vi "TombOfTheMask.vi"() -> ()   [LabVIEW 2014]
panel:
  out "stage":dbl
  in  "start":cluster{"String":string, "play":bool}={"String"="\nTomb Of The Mask", "play"=FALSE}
  in  "quit":bool
  in  "next stage or choosing stage":T1
  in  "choosing stage":T2
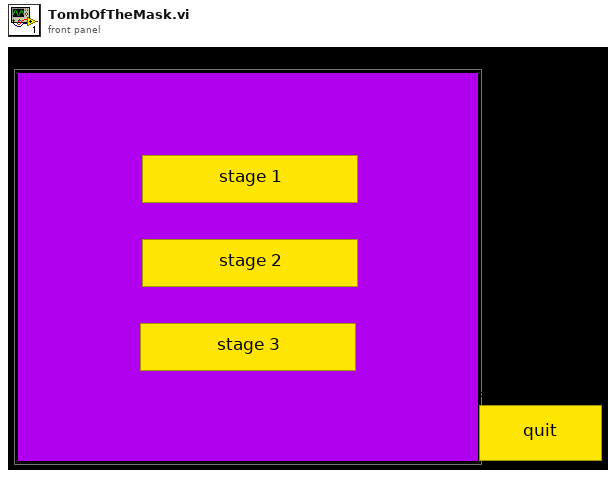
[diagram p1: front panel]
types:
  T1 = cluster{"next stage ":bool, "back":bool, "Boolean":bool, "Boolean 2":bool, "Boolean 3":bool}
  T2 = cluster{"stage 1":bool, "stage 2":bool, "stsage 3":bool}
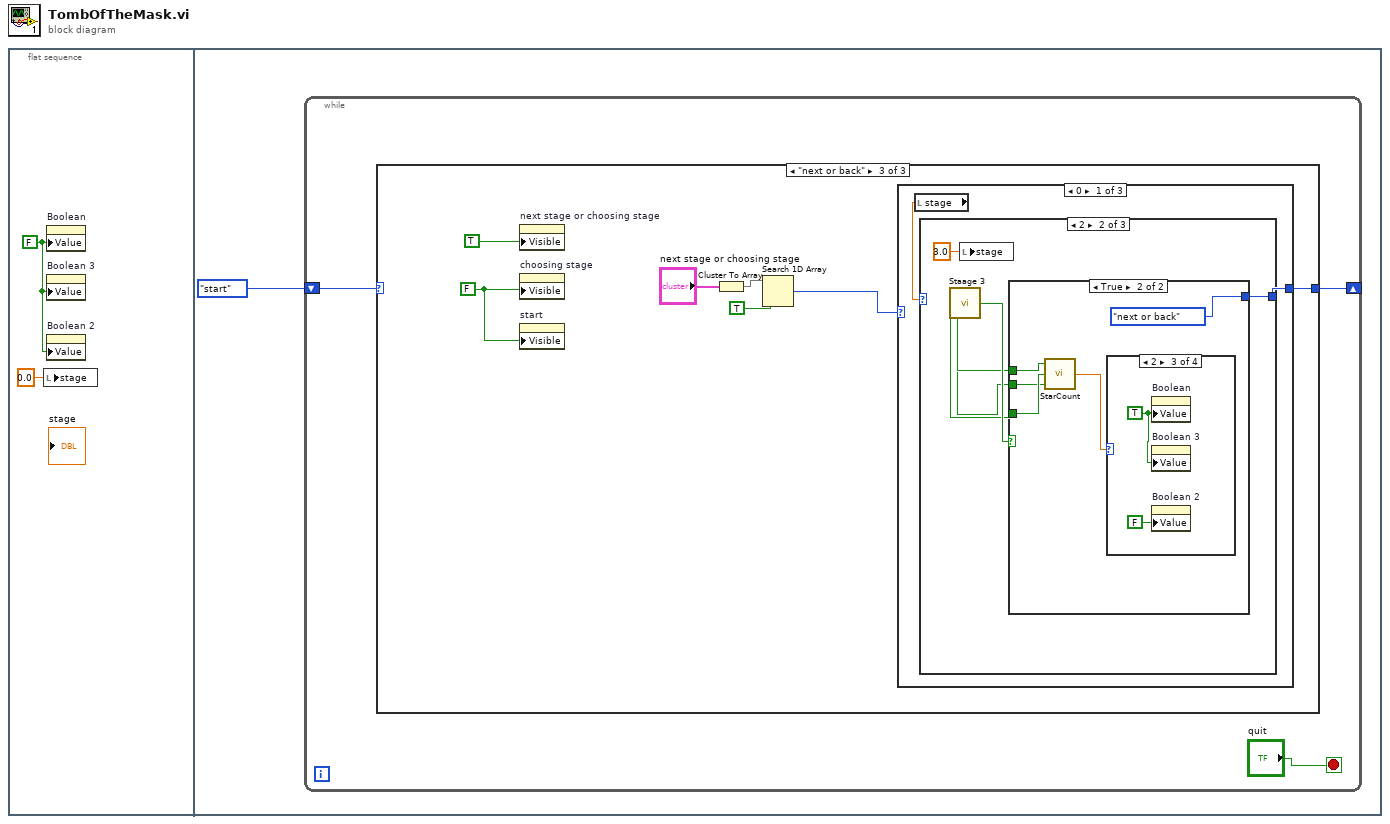
[diagram p0: block diagram]
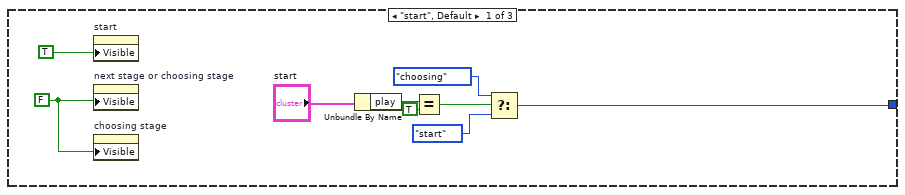
[diagram p2: hidden frame]
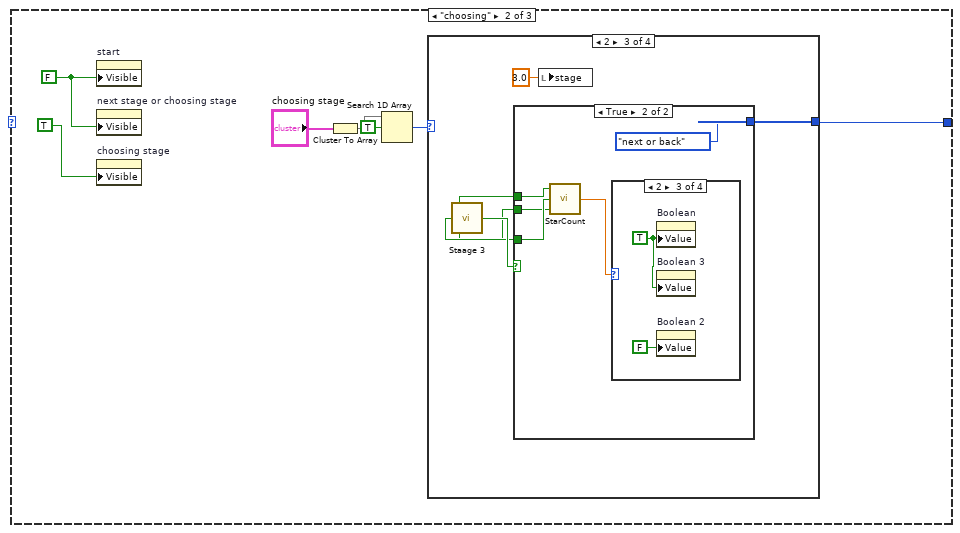
[diagram p3: hidden frame]
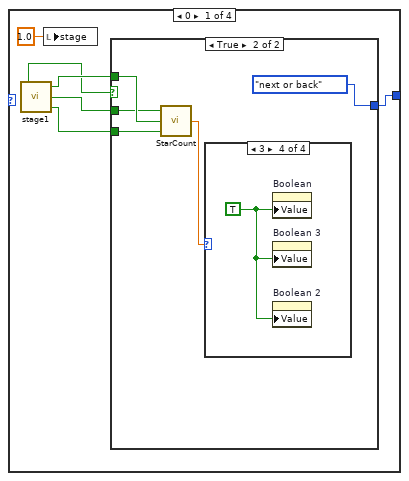
[diagram p4: hidden frame]
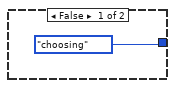
[diagram p5: hidden frame]
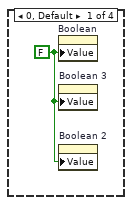
[diagram p6: hidden frame]
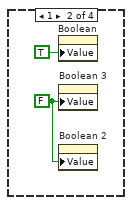
[diagram p7: hidden frame]
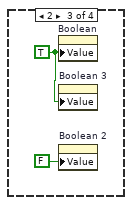
[diagram p8: hidden frame]
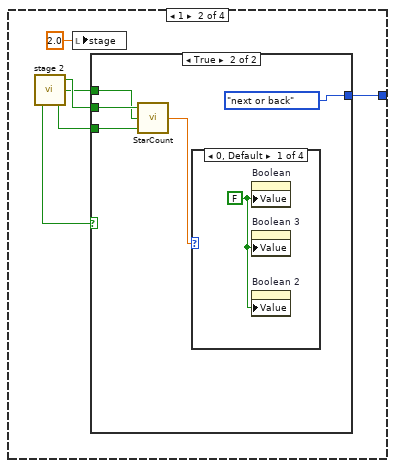
[diagram p9: hidden frame]
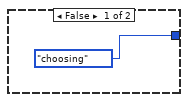
[diagram p10: hidden frame]
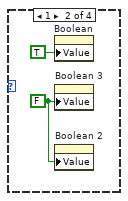
[diagram p11: hidden frame]
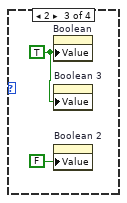
[diagram p12: hidden frame]
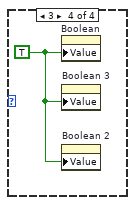
[diagram p13: hidden frame]
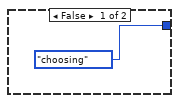
[diagram p14: hidden frame]
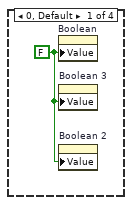
[diagram p15: hidden frame]
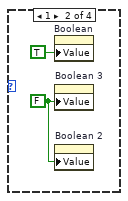
[diagram p16: hidden frame]
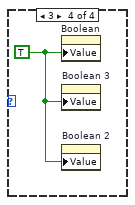
[diagram p17: hidden frame]
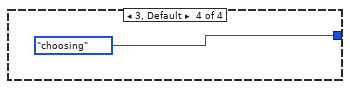
[diagram p18: hidden frame]
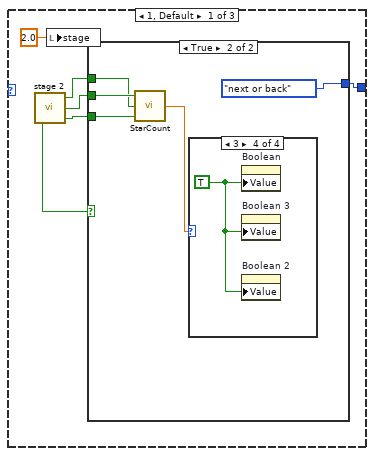
[diagram p19: hidden frame]
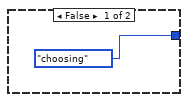
[diagram p20: hidden frame]
diagram:
  n1 = flat-sequence {
    frame #0 {
      w1 = FALSE ("Value")
      n2 = local write "stage"(0.0 ("stage")) -> ()
      n3 = property on="Boolean" class="Bool (strict)"("Value"=w1) -> ()  [unwired: 2 in, 2 out]
      n4 = property on="Boolean 3" class="Bool (strict)"("Value"=w1) -> ()  [unwired: 2 in, 2 out]
      n5 = property on="Boolean 2" class="Bool (strict)"("Value"=w1) -> ()  [unwired: 2 in, 2 out]
    }
    frame #1 {
      n6 = while {
        shift-right: [w5] -> _
        shift-left: enum16{"next or back", "choosing", "start"}."start" ("Enum") -> [w6]
        stop <- "quit" stop-if-true
        n7 = case shown="\"next or back\"" w6 {
          tunnel: [w7 w16 w78] -> w5
          frame "start", Default {
            w14 = FALSE ("Visible")
            n8 = property on="start" class="Clust"("Visible"=TRUE) -> ()  [unwired: 2 in, 2 out]
            n9 = property on="next stage or choosing stage" class="Clust"("Visible"=w14) -> ()  [unwired: 2 in, 2 out]
            n10 = property on="choosing stage" class="Clust"("Visible"=w14) -> ()  [unwired: 2 in, 2 out]
            n11 = Unbundle By Name("start") -> ("play"=w12:bool)
            n12 = Equal?(x=w12, y=TRUE) -> (x = y?=w10:bool)
            n13 = Select(t=enum16{"next or back", "choosing", "start"}."choosing" ("Enum"), s=w10, f=enum16{"next or back", "choosing", "start"}."start" ("Enum")) -> (s? t:f=w7:enum16{"next or back", "choosing", "start"})
          }
          frame "choosing" {
            w21 = FALSE ("Visible")
            n14 = property on="start" class="Clust"("Visible"=w21) -> ()  [unwired: 2 in, 2 out]
            n15 = property on="next stage or choosing stage" class="Clust"("Visible"=w21) -> ()  [unwired: 2 in, 2 out]
            n16 = property on="choosing stage" class="Clust"("Visible"=TRUE) -> ()  [unwired: 2 in, 2 out]
            n17 = Cluster To Array(cluster="choosing stage") -> (array=w19:bool[])
            n18 = Search 1D Array(1D array=w19, element=TRUE) -> (index of element=w17:i32)  [unwired: 1 in]
            n19 = case shown="2" w17 {
              tunnel: [w25 w41 w59 enum16{"next or back", "choosing", "start"}."choosing" ("Enum")] -> w16
              frame 0 {
                n20 = call "stage1.vi"() -> ("pass"=w24:bool, "Boolean 5"=w26:bool, "Boolean 8"=w23:bool, "Boolean 7"=w27:bool)
                n21 = local write "stage"(1.0 ("stage")) -> ()
                n22 = case shown="True" w24 {
                  tunnel: w27 -> [_ w34]
                  tunnel: w26 -> [_ w33]
                  tunnel: w23 -> [_ w32]
                  tunnel: [enum16{"next or back", "choosing", "start"}."choosing" ("Enum") enum16{"next or back", "choosing", "start"}."next or back" ("Enum")] -> w25
                  frame False {
                  }
                  frame True {
                    n23 = call "StarCount.vi"("Boolean 2"=w34, "Boolean"=w33, "Boolean 3"=w32) -> ("Numeric"=w30:dbl)
                    n24 = case shown="3" w30 {
                      frame 0, Default {
                        w35 = FALSE ("Value")
                        n25 = property on="Boolean" class="Bool (strict)"("Value"=w35) -> ()  [unwired: 2 in, 2 out]
                        n26 = property on="Boolean 3" class="Bool (strict)"("Value"=w35) -> ()  [unwired: 2 in, 2 out]
                        n27 = property on="Boolean 2" class="Bool (strict)"("Value"=w35) -> ()  [unwired: 2 in, 2 out]
                      }
                      frame 1 {
                        w36 = FALSE ("Value")
                        n28 = property on="Boolean" class="Bool (strict)"("Value"=TRUE) -> ()  [unwired: 2 in, 2 out]
                        n29 = property on="Boolean 3" class="Bool (strict)"("Value"=w36) -> ()  [unwired: 2 in, 2 out]
                        n30 = property on="Boolean 2" class="Bool (strict)"("Value"=w36) -> ()  [unwired: 2 in, 2 out]
                      }
                      frame 2 {
                        w39 = TRUE ("Value")
                        n31 = property on="Boolean" class="Bool (strict)"("Value"=w39) -> ()  [unwired: 2 in, 2 out]
                        n32 = property on="Boolean 3" class="Bool (strict)"("Value"=w39) -> ()  [unwired: 2 in, 2 out]
                        n33 = property on="Boolean 2" class="Bool (strict)"("Value"=FALSE) -> ()  [unwired: 2 in, 2 out]
                      }
                      frame 3 {
                        w40 = TRUE ("Value")
                        n34 = property on="Boolean" class="Bool (strict)"("Value"=w40) -> ()  [unwired: 2 in, 2 out]
                        n35 = property on="Boolean 3" class="Bool (strict)"("Value"=w40) -> ()  [unwired: 2 in, 2 out]
                        n36 = property on="Boolean 2" class="Bool (strict)"("Value"=w40) -> ()  [unwired: 2 in, 2 out]
                      }
                    }
                  }
                }
              }
              frame 1 {
                n37 = call "stage 2.vi"() -> ("pass"=w45:bool, "Boolean 5"=w44:bool, "Boolean 7"=w43:bool, "Boolean 8"=w42:bool)
                n38 = local write "stage"(2.0 ("stage")) -> ()
                n39 = case shown="True" w45 {
                  tunnel: w44 -> [_ w52]
                  tunnel: w43 -> [_ w51]
                  tunnel: w42 -> [_ w50]
                  tunnel: [enum16{"next or back", "choosing", "start"}."choosing" ("Enum") enum16{"next or back", "choosing", "start"}."next or back" ("Enum")] -> w41
                  frame False {
                  }
                  frame True {
                    n40 = call "StarCount.vi"("Boolean 2"=w50, "Boolean"=w51, "Boolean 3"=w52) -> ("Numeric"=w49:dbl)
                    n41 = case shown="0, Default" w49 {
                      frame 0, Default {
                        w53 = FALSE ("Value")
                        n42 = property on="Boolean" class="Bool (strict)"("Value"=w53) -> ()  [unwired: 2 in, 2 out]
                        n43 = property on="Boolean 3" class="Bool (strict)"("Value"=w53) -> ()  [unwired: 2 in, 2 out]
                        n44 = property on="Boolean 2" class="Bool (strict)"("Value"=w53) -> ()  [unwired: 2 in, 2 out]
                      }
                      frame 1 {
                        w54 = FALSE ("Value")
                        n45 = property on="Boolean" class="Bool (strict)"("Value"=TRUE) -> ()  [unwired: 2 in, 2 out]
                        n46 = property on="Boolean 3" class="Bool (strict)"("Value"=w54) -> ()  [unwired: 2 in, 2 out]
                        n47 = property on="Boolean 2" class="Bool (strict)"("Value"=w54) -> ()  [unwired: 2 in, 2 out]
                      }
                      frame 2 {
                        w57 = TRUE ("Value")
                        n48 = property on="Boolean" class="Bool (strict)"("Value"=w57) -> ()  [unwired: 2 in, 2 out]
                        n49 = property on="Boolean 3" class="Bool (strict)"("Value"=w57) -> ()  [unwired: 2 in, 2 out]
                        n50 = property on="Boolean 2" class="Bool (strict)"("Value"=FALSE) -> ()  [unwired: 2 in, 2 out]
                      }
                      frame 3 {
                        w58 = TRUE ("Value")
                        n51 = property on="Boolean" class="Bool (strict)"("Value"=w58) -> ()  [unwired: 2 in, 2 out]
                        n52 = property on="Boolean 3" class="Bool (strict)"("Value"=w58) -> ()  [unwired: 2 in, 2 out]
                        n53 = property on="Boolean 2" class="Bool (strict)"("Value"=w58) -> ()  [unwired: 2 in, 2 out]
                      }
                    }
                  }
                }
              }
              frame 2 {
                n54 = call "Staage 3.vi"() -> ("pass"=w63:bool, "Boolean 5"=w60:bool, "Boolean 7"=w61:bool, "Boolean 8"=w62:bool)
                n55 = case shown="True" w63 {
                  tunnel: w62 -> [_ w70]
                  tunnel: w61 -> [_ w69]
                  tunnel: w60 -> [_ w68]
                  tunnel: [enum16{"next or back", "choosing", "start"}."choosing" ("Enum") enum16{"next or back", "choosing", "start"}."next or back" ("Enum")] -> w59
                  frame False {
                  }
                  frame True {
                    n56 = call "StarCount.vi"("Boolean 2"=w68, "Boolean"=w69, "Boolean 3"=w70) -> ("Numeric"=w67:dbl)
                    n57 = case shown="2" w67 {
                      frame 0, Default {
                        w71 = FALSE ("Value")
                        n58 = property on="Boolean" class="Bool (strict)"("Value"=w71) -> ()  [unwired: 2 in, 2 out]
                        n59 = property on="Boolean 3" class="Bool (strict)"("Value"=w71) -> ()  [unwired: 2 in, 2 out]
                        n60 = property on="Boolean 2" class="Bool (strict)"("Value"=w71) -> ()  [unwired: 2 in, 2 out]
                      }
                      frame 1 {
                        w72 = FALSE ("Value")
                        n61 = property on="Boolean" class="Bool (strict)"("Value"=TRUE) -> ()  [unwired: 2 in, 2 out]
                        n62 = property on="Boolean 3" class="Bool (strict)"("Value"=w72) -> ()  [unwired: 2 in, 2 out]
                        n63 = property on="Boolean 2" class="Bool (strict)"("Value"=w72) -> ()  [unwired: 2 in, 2 out]
                      }
                      frame 2 {
                        w75 = TRUE ("Value")
                        n64 = property on="Boolean" class="Bool (strict)"("Value"=w75) -> ()  [unwired: 2 in, 2 out]
                        n65 = property on="Boolean 3" class="Bool (strict)"("Value"=w75) -> ()  [unwired: 2 in, 2 out]
                        n66 = property on="Boolean 2" class="Bool (strict)"("Value"=FALSE) -> ()  [unwired: 2 in, 2 out]
                      }
                      frame 3 {
                        w76 = TRUE ("Value")
                        n67 = property on="Boolean" class="Bool (strict)"("Value"=w76) -> ()  [unwired: 2 in, 2 out]
                        n68 = property on="Boolean 3" class="Bool (strict)"("Value"=w76) -> ()  [unwired: 2 in, 2 out]
                        n69 = property on="Boolean 2" class="Bool (strict)"("Value"=w76) -> ()  [unwired: 2 in, 2 out]
                      }
                    }
                  }
                }
                n70 = local write "stage"(3.0 ("stage")) -> ()
              }
              frame 3, Default {
              }
            }
          }
          frame "next or back" {
            w83 = FALSE ("Visible")
            n71 = property on="next stage or choosing stage" class="Clust"("Visible"=TRUE) -> ()  [unwired: 2 in, 2 out]
            n72 = property on="choosing stage" class="Clust"("Visible"=w83) -> ()  [unwired: 2 in, 2 out]
            n73 = property on="start" class="Clust"("Visible"=w83) -> ()  [unwired: 2 in, 2 out]
            n74 = Cluster To Array(cluster="next stage or choosing stage") -> (array=w81:bool[])
            n75 = Search 1D Array(1D array=w81, element=TRUE) -> (index of element=w79:i32)  [unwired: 1 in]
            n76 = case shown="0" w79 {
              tunnel: [w85 enum16{"next or back", "choosing", "start"}."choosing" ("Enum") enum16{"next or back", "choosing", "start"}."next or back" ("Enum")] -> w78
              frame 0 {
                n77 = local read "stage"() -> (w86:dbl)
                n78 = case shown="2" w86 {
                  tunnel: [w88 w110 enum16{"next or back", "choosing", "start"}."start" ("Enum")] -> w85
                  frame 1, Default {
                    n79 = call "stage 2.vi"() -> ("pass"=w92:bool, "Boolean 5"=w91:bool, "Boolean 7"=w90:bool, "Boolean 8"=w89:bool)
                    n80 = local write "stage"(2.0 ("stage")) -> ()
                    n81 = case shown="True" w92 {
                      tunnel: w90 -> [_ w98]
                      tunnel: w91 -> [_ w97]
                      tunnel: w89 -> [_ w96]
                      tunnel: [enum16{"next or back", "choosing", "start"}."choosing" ("Enum") enum16{"next or back", "choosing", "start"}."next or back" ("Enum")] -> w88
                      frame False {
                      }
                      frame True {
                        n82 = call "StarCount.vi"("Boolean 2"=w96, "Boolean"=w97, "Boolean 3"=w98) -> ("Numeric"=w95:dbl)
                        n83 = case shown="3" w95 {
                          frame 0, Default {
                            w99 = FALSE ("Value")
                            n84 = property on="Boolean" class="Bool (strict)"("Value"=w99) -> ()  [unwired: 2 in, 2 out]
                            n85 = property on="Boolean 3" class="Bool (strict)"("Value"=w99) -> ()  [unwired: 2 in, 2 out]
                            n86 = property on="Boolean 2" class="Bool (strict)"("Value"=w99) -> ()  [unwired: 2 in, 2 out]
                          }
                          frame 1 {
                            w100 = FALSE ("Value")
                            n87 = property on="Boolean" class="Bool (strict)"("Value"=TRUE) -> ()  [unwired: 2 in, 2 out]
                            n88 = property on="Boolean 3" class="Bool (strict)"("Value"=w100) -> ()  [unwired: 2 in, 2 out]
                            n89 = property on="Boolean 2" class="Bool (strict)"("Value"=w100) -> ()  [unwired: 2 in, 2 out]
                          }
                          frame 2 {
                            w103 = TRUE ("Value")
                            n90 = property on="Boolean" class="Bool (strict)"("Value"=w103) -> ()  [unwired: 2 in, 2 out]
                            n91 = property on="Boolean 3" class="Bool (strict)"("Value"=w103) -> ()  [unwired: 2 in, 2 out]
                            n92 = property on="Boolean 2" class="Bool (strict)"("Value"=FALSE) -> ()  [unwired: 2 in, 2 out]
                          }
                          frame 3 {
                            w104 = TRUE ("Value")
                            n93 = property on="Boolean" class="Bool (strict)"("Value"=w104) -> ()  [unwired: 2 in, 2 out]
                            n94 = property on="Boolean 3" class="Bool (strict)"("Value"=w104) -> ()  [unwired: 2 in, 2 out]
                            n95 = property on="Boolean 2" class="Bool (strict)"("Value"=w104) -> ()  [unwired: 2 in, 2 out]
                          }
                        }
                      }
                    }
                  }
                  frame 2 {
                    n96 = call "Staage 3.vi"() -> ("pass"=w109:bool, "Boolean 5"=w106:bool, "Boolean 7"=w107:bool, "Boolean 8"=w108:bool)
                    n97 = local write "stage"(3.0 ("stage")) -> ()
                    n98 = case shown="True" w109 {
                      tunnel: [enum16{"next or back", "choosing", "start"}."choosing" ("Enum") enum16{"next or back", "choosing", "start"}."next or back" ("Enum")] -> w110
                      tunnel: w108 -> [_ w114]
                      tunnel: w107 -> [_ w113]
                      tunnel: w106 -> [_ w112]
                      frame False {
                      }
                      frame True {
                        n99 = call "StarCount.vi"("Boolean 2"=w112, "Boolean"=w113, "Boolean 3"=w114) -> ("Numeric"=w116:dbl)
                        n100 = case shown="2" w116 {
                          frame 0, Default {
                            w117 = FALSE ("Value")
                            n101 = property on="Boolean" class="Bool (strict)"("Value"=w117) -> ()  [unwired: 2 in, 2 out]
                            n102 = property on="Boolean 3" class="Bool (strict)"("Value"=w117) -> ()  [unwired: 2 in, 2 out]
                            n103 = property on="Boolean 2" class="Bool (strict)"("Value"=w117) -> ()  [unwired: 2 in, 2 out]
                          }
                          frame 1 {
                            w118 = FALSE ("Value")
                            n104 = property on="Boolean" class="Bool (strict)"("Value"=TRUE) -> ()  [unwired: 2 in, 2 out]
                            n105 = property on="Boolean 3" class="Bool (strict)"("Value"=w118) -> ()  [unwired: 2 in, 2 out]
                            n106 = property on="Boolean 2" class="Bool (strict)"("Value"=w118) -> ()  [unwired: 2 in, 2 out]
                          }
                          frame 2 {
                            w121 = TRUE ("Value")
                            n107 = property on="Boolean" class="Bool (strict)"("Value"=w121) -> ()  [unwired: 2 in, 2 out]
                            n108 = property on="Boolean 3" class="Bool (strict)"("Value"=w121) -> ()  [unwired: 2 in, 2 out]
                            n109 = property on="Boolean 2" class="Bool (strict)"("Value"=FALSE) -> ()  [unwired: 2 in, 2 out]
                          }
                          frame 3 {
                            w122 = TRUE ("Value")
                            n110 = property on="Boolean" class="Bool (strict)"("Value"=w122) -> ()  [unwired: 2 in, 2 out]
                            n111 = property on="Boolean 3" class="Bool (strict)"("Value"=w122) -> ()  [unwired: 2 in, 2 out]
                            n112 = property on="Boolean 2" class="Bool (strict)"("Value"=w122) -> ()  [unwired: 2 in, 2 out]
                          }
                        }
                      }
                    }
                  }
                  frame 3 {
                  }
                }
              }
              frame 1 {
              }
              frame 2, Default {
              }
            }
          }
        }
      }
    }
  }
